vi "4. Find Words.vi"() -> ()   [LabVIEW 2020]
panel:
  out "Array":string[](array[string])
  in  "String Array":string[](array[string])
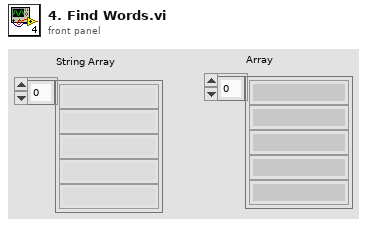
[diagram p1: front panel]
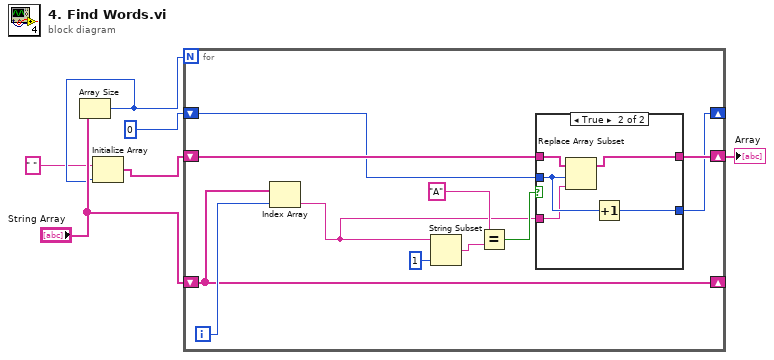
[diagram p0: block diagram]
diagram:
  n1 = Array Size(array="String Array") -> (size(s)=w3:i32)
  n2 = Initialize Array "Initialize Array"(" ", w3) -> (w4:string[])
  n3 = for {
    N: w3 -> [_]
    shift-right: [w15] -> _
    shift-left: "String Array" -> [w15]
    shift-right: [w10] -> w1
    shift-left: w4 -> [w12]
    shift-right: [w8] -> _
    shift-left: 0 -> [w11]
    i -> [w17]
    n4 = Index Array "Index Array"(array=w15, index=w17) -> (element=w7:string)
    n5 = String Subset(string=w7, length (rest)=1 ("length (rest)")) -> (substring=w9:string)  [unwired: 1 in]
    n6 = Equal?(x="A", y=w9) -> (x = y?=w13:bool)
    n7 = case shown="True" w13 {
      tunnel: w12 -> [w18 w24]
      tunnel: w11 -> [w19 w22]
      tunnel: [w18 w23] -> w10
      tunnel: [w19 w21] -> w8
      tunnel: w7 -> [_ w20]
      frame False {
      }
      frame True {
        n8 = Replace Array Subset "Replace Array Subset"(array=w24, new element=w20, index=w22) -> (w23:string[])
        n9 = Increment(x=w22) -> (x+1=w21:i32)
      }
    }
  }
  "Array" <- w1
